vi "standard frame scan geometry_grMD.vi"() -> (3 "frame scan geometry out":waveform(dbl)[](array[waveform]))   [LabVIEW 2017]
doc: "SciScan 1.2 160622"
uses:
  <vilib>/Analysis/coordinate.llb/2D Cartesian Coordinate Rotation (Array).vi
  GFG/GFGnumericGet.vi
  GFG/GFGbooleanGet.vi
  GFG/GFG library.lvlib
  <vilib>/Analysis/NI_AALPro.lvlib
panel:
  out "x waveform":waveform(dbl)
  out "y waveform":waveform(dbl)
  out "Waveform Graph 2":waveform(dbl)(graph)
  out "Waveform Graph":waveform(dbl)(graph)
  out "y waveform (two frames)":dbl[](array[numeric])
  out "x waveform (two frames)":dbl[](array[numeric])
  out "XY Graph":cluster{"Y":dbl[], "Y":dbl[]}[](graph)
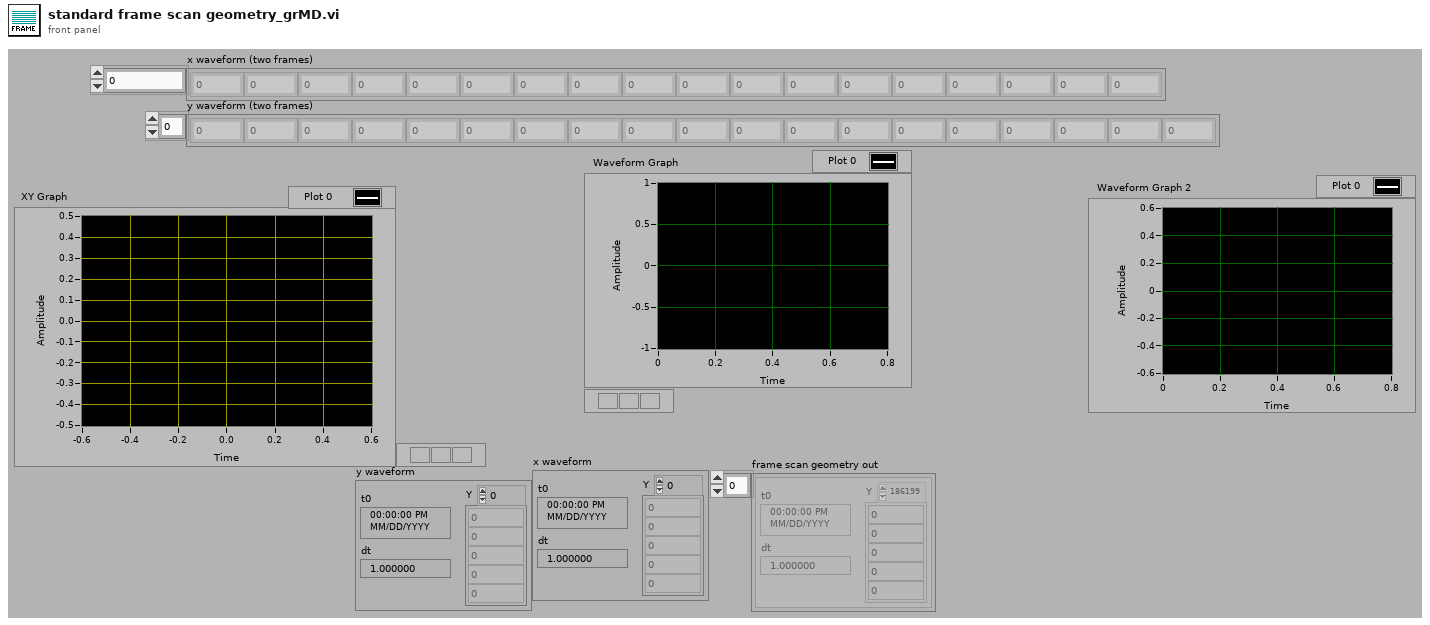
[diagram p1: front panel]
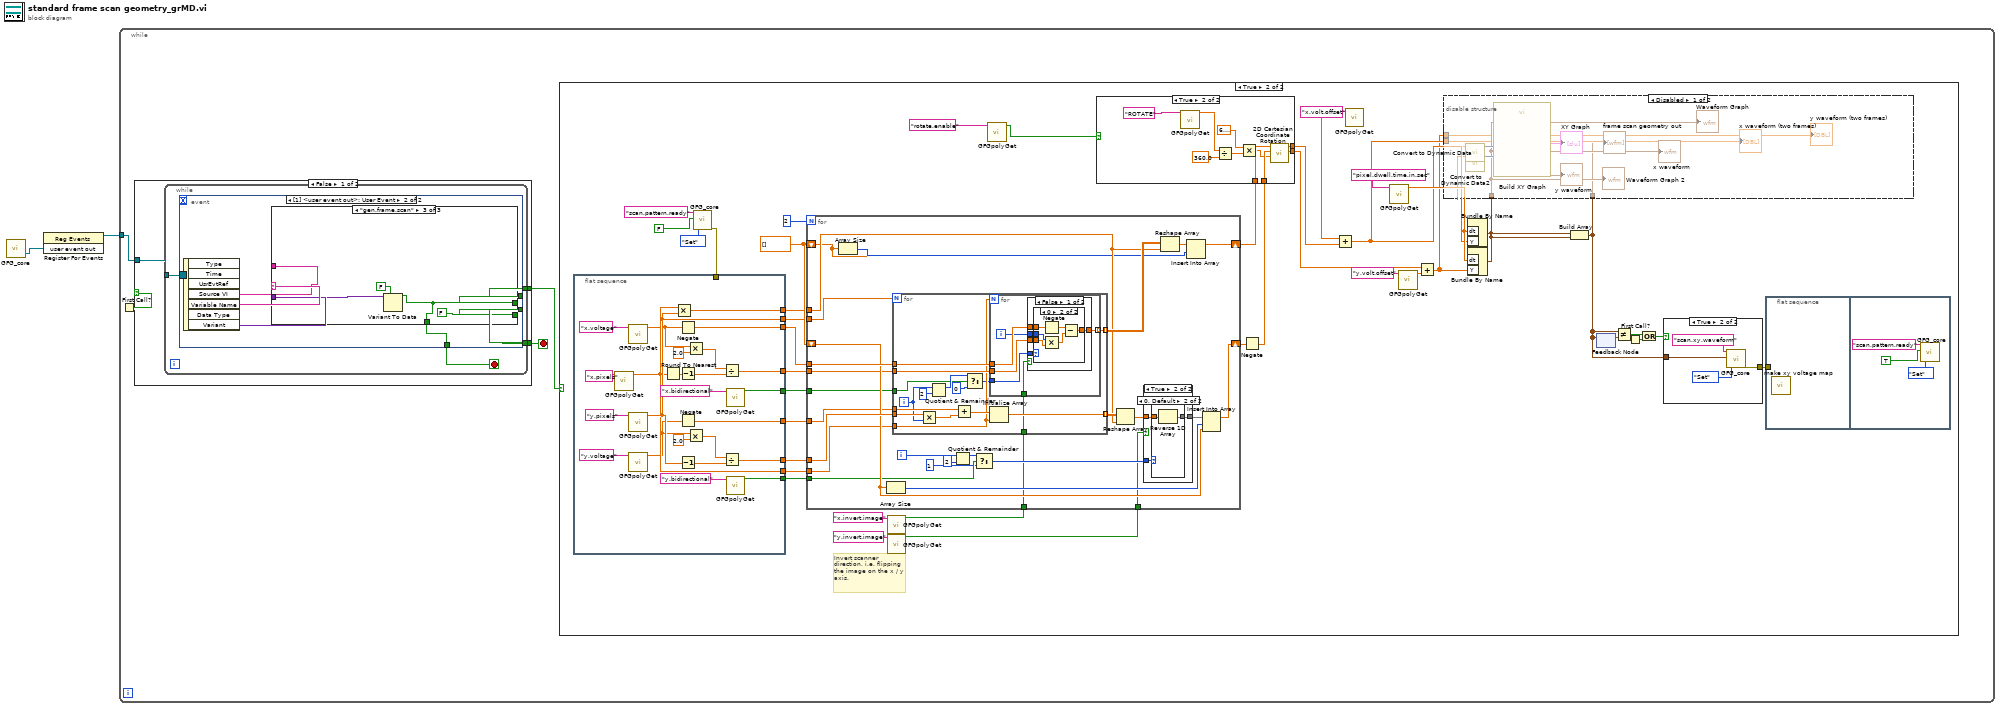
[diagram p0: block diagram]
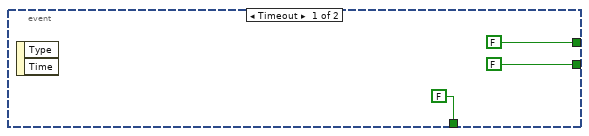
[diagram p2: hidden frame]
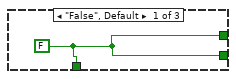
[diagram p3: hidden frame]
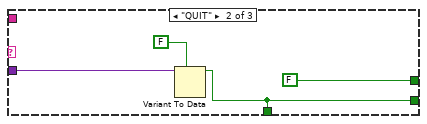
[diagram p4: hidden frame]
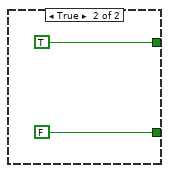
[diagram p5: hidden frame]
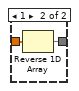
[diagram p11: hidden frame]
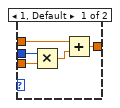
[diagram p13: hidden frame]
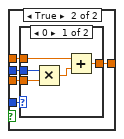
[diagram p14: hidden frame]
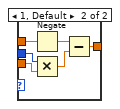
[diagram p15: hidden frame]
diagram:
  n1 = call "GFG_core.vi"() -> ("user event out"=w2:refnum<user-event>)  [unwired: 13 in, 6 out]
  n2 = register-events(w2) -> (reference out=w1:refnum<event-registration>)  [unwired: 2 in, 1 out]
  n3 = while {
    tunnel: w1 -> [w6]
    stop <- w5 stop-if-true
    n4 = First Call?() -> (First Call?: T/F=w3:bool)
    n5 = case shown="False" w3 {
      tunnel: w6 -> [w9 _]
      tunnel: [w8 FALSE ("NewVal")] -> w5
      tunnel: [w7 TRUE ("NewVal")] -> w4
      frame False {
        n6 = while {
          tunnel: w9 -> [w13]
          tunnel: [w11] -> w8
          tunnel: [w12] -> w7
          stop <- w10 stop-if-true
          n7 = event shown="[1] <user event out>: User Event" {
            selector: w13 -> [_ _]
            dyn-events: _ -> [_ _]
            timeout: _ -> [_ _]
            tunnel: [FALSE ("NewVal") w21] -> w12
            tunnel: [FALSE ("NewVal") w20] -> w11
            tunnel: [FALSE w18] -> w10
            event Timeout {
              n8 = event-data() -> ()  [unwired: 1 in, 2 out]
            }
            event User Event {
              n9 = event-data() -> ("Source VI"=w17:string, "Variable Name"=w22:string, "Variant"=w19:variant)  [unwired: 1 in, 4 out]
              n10 = case shown="\"gen.frame.scan\"" w22 {
                tunnel: [w23 FALSE ("NewVal") w28] -> w21
                tunnel: [w23 w24 FALSE] -> w20
                tunnel: w19 -> [_ w27 w29]
                tunnel: [w23 w24 w28] -> w18
                tunnel: w17 -> [_ _ _]
                frame "False", Default {
                  w23 = FALSE ("NewVal")
                }
                frame "QUIT" {
                  n11 = Variant To Data(type=FALSE ("NewVal"), Variant=w27) -> (data=w24:bool)  [unwired: 1 in, 1 out]
                }
                frame "gen.frame.scan" {
                  n12 = Variant To Data(type=FALSE ("NewVal"), Variant=w29) -> (data=w28:bool)  [unwired: 1 in, 1 out]
                }
              }
            }
          }
        }
      }
      frame True {
      }
    }
    n13 = case shown="True" w4 {
      frame False {
      }
      frame True {
        w72 = dbl[] []
        # "Invert scanner direction, i.e. flipping the image on the x / y axis."
        n14 = flat-sequence {
          tunnel: [w109] -> w75
          tunnel: [w108] -> w74
          tunnel: [w106] -> w71
          tunnel: [w102] -> w70
          tunnel: [w101] -> w69
          tunnel: [w100] -> w68
          tunnel: [w98] -> w67
          tunnel: [w92] -> w66
          tunnel: [w90] -> w65
          tunnel: w46 -> [_]
          frame #0 {
            n15 = call-poly "GFGpolyGet.vi"("Variable Name in"="x.pixels" ("Tag in")) -> ("Numeric"=w98:dbl)  [unwired: 8 in, 2 out]
            n16 = call-poly "GFGpolyGet.vi"("Variable Name in"="x.voltage" ("Tag in")) -> ("Numeric"=w96:dbl)  [unwired: 8 in, 2 out]
            n17 = call-poly "GFGpolyGet.vi"("Variable Name in"="y.pixels" ("Tag in")) -> ("Numeric"=w100:dbl)  [unwired: 8 in, 2 out]
            n18 = call-poly "GFGpolyGet.vi"("Variable Name in"="y.voltage" ("Tag in")) -> ("Numeric"=w94:dbl)  [unwired: 8 in, 2 out]
            n19 = Round To Nearest(number=w98) -> (nearest integer value=w88:dbl)
            n20 = Multiply(x=w98, y=w100) -> (x*y=w101:dbl)
            n21 = Negate(x=w96) -> (-x=w109:dbl)
            n22 = Decrement(x=w88) -> (x-1=w105:dbl)
            n23 = Negate(x=w94) -> (-x=w106:dbl)
            n24 = Decrement(x=w100) -> (x-1=w107:dbl)
            n25 = Multiply(x=w96, y=2.0) -> (x*y=w104:dbl)
            n26 = Multiply(x=w94, y=2.0) -> (x*y=w110:dbl)
            n27 = Divide(x=w104, y=w105) -> (x/y=w102:dbl)
            n28 = Divide(x=w110, y=w107) -> (x/y=w108:dbl)
            n29 = call-poly "GFGpolyGet.vi"("Variable Name in"="x.bidirectional" ("Tag in")) -> ("Boolean Value OUT"=w90:bool)  [unwired: 9 in, 1 out]
            n30 = call-poly "GFGpolyGet.vi"("Variable Name in"="y.bidirectional" ("Tag in")) -> ("Boolean Value OUT"=w92:bool)  [unwired: 9 in, 1 out]
          }
        }
        n31 = call "GFG_core.vi"("Variable Name in"="scan.pattern.ready", "Variant in"=FALSE, "Action"=enum16{"Init", "Set", "Get"}."Set") -> ("error out"=w46:errorcluster)  [unwired: 10 in, 6 out]
        n32 = call-poly "GFGpolyGet.vi"("Variable Name in"="x.invert.image" ("Tag in")) -> ("Boolean Value OUT"=w34:bool)  [unwired: 9 in, 1 out]
        n33 = call-poly "GFGpolyGet.vi"("Variable Name in"="y.invert.image" ("Tag in")) -> ("Boolean Value OUT"=w35:bool)  [unwired: 9 in, 1 out]
        n34 = for {
          N: 2 -> [_]
          tunnel: w75 -> [w153]
          tunnel: w74 -> [w152]
          tunnel: w68 -> [w136]
          tunnel: w69 -> [w149]
          shift-right: [w144] -> w38
          shift-left: w72 -> [w146]
          shift-right: [w140] -> w37
          shift-left: w72 -> [w142]
          tunnel: w67 -> [w139]
          tunnel: w71 -> [w138]
          tunnel: w70 -> [w137]
          tunnel: w66 -> [w132]
          tunnel: w65 -> [w131]
          tunnel: w35 -> [w127]
          tunnel: w34 -> [w128]
          i -> [w130]
          n35 = Array Size(array=w146) -> (size(s)=w147:i32)
          n36 = Array Size(array=w142) -> (size(s)=w141:i32)
          n37 = for {
            N: w136 -> [_]
            tunnel: w139 -> [w173]
            tunnel: w153 -> [w175]
            tunnel: w152 -> [w181]
            tunnel: [w178] -> w151 mode=indexing
            tunnel: [w177] -> w150 mode=indexing
            tunnel: w138 -> [w176]
            tunnel: w137 -> [w174]
            tunnel: w131 -> [w167]
            tunnel: w128 -> [w166]
            i -> [w169]
            n38 = Multiply(x=w181, y=w169) -> (x*y=w180:dbl)
            n39 = Quotient & Remainder(x=w169, y=2) -> (x-y*floor(x/y)=w172:i32)  [unwired: 1 out]
            n40 = Add(x=w176, y=w180) -> (x+y=w179:dbl)
            n41 = Select(t=w172, s=w167, f=0) -> (s? t:f=w168:i32)
            n42 = for {
              N: w173 -> [_]
              tunnel: w174 -> [w187]
              tunnel: [w186] -> w178 mode=indexing
              tunnel: w175 -> [w185]
              tunnel: w168 -> [w183]
              tunnel: w166 -> [w182]
              i -> [w184]
              n43 = case shown="False" w182 {
                tunnel: w187 -> [w192 w206]
                tunnel: [w191 w205] -> w186
                tunnel: w185 -> [w190 w208]
                tunnel: w184 -> [w189 w207]
                tunnel: w183 -> [w188 w204]
                frame False {
                  n44 = case shown="0" w188 {
                    tunnel: w192 -> [w197 w203]
                    tunnel: [w196 w202] -> w191
                    tunnel: w190 -> [w195 w201]
                    tunnel: w189 -> [w193 w199]
                    frame 1, Default {
                      n45 = Multiply(x=w193, y=w197) -> (x*y=w194:dbl)
                      n46 = Add(x=w195, y=w194) -> (x+y=w196:dbl)
                    }
                    frame 0 {
                      n47 = Negate(x=w201) -> (-x=w198:dbl)
                      n48 = Multiply(x=w199, y=w203) -> (x*y=w200:dbl)
                      n49 = Subtract(x=w198, y=w200) -> (x-y=w202:dbl)
                    }
                  }
                }
                frame True {
                  n50 = case shown="0" w204 {
                    tunnel: w206 -> [w213 w219]
                    tunnel: [w212 w218] -> w205
                    tunnel: w208 -> [w211 w217]
                    tunnel: w207 -> [w209 w215]
                    frame 0 {
                      n51 = Multiply(x=w209, y=w213) -> (x*y=w210:dbl)
                      n52 = Add(x=w211, y=w210) -> (x+y=w212:dbl)
                    }
                    frame 1, Default {
                      n53 = Negate(x=w217) -> (-x=w214:dbl)
                      n54 = Multiply(x=w215, y=w219) -> (x*y=w216:dbl)
                      n55 = Subtract(x=w214, y=w216) -> (x-y=w218:dbl)
                    }
                  }
                }
              }
            }
            n56 = Initialize Array(w179, w173) -> (w177:dbl[])
          }
          n57 = Quotient & Remainder(x=w130, y=2) -> (x-y*floor(x/y)=w134:i32)  [unwired: 1 out]
          n58 = Select(t=w134, s=w132, f=1) -> (s? t:f=w133:i32)
          n59 = Reshape Array(w150, w149) -> (w148:dbl[])
          n60 = case shown="True" w127 {
            tunnel: w148 -> [w156 w162]
            tunnel: [w155 w161] -> w143
            tunnel: w133 -> [w154 w160]
            frame False {
              n61 = case shown="0, Default" w154 {
                tunnel: [w157 w158] -> w155
                tunnel: w156 -> [w157 w159]
                frame 0, Default {
                }
                frame 1 {
                  n62 = Reverse 1D Array(array=w159) -> (reversed array=w158:dbl[])
                }
              }
            }
            frame True {
              n63 = case shown="0, Default" w160 {
                tunnel: [w163 w164] -> w161
                tunnel: w162 -> [w163 w165]
                frame 1 {
                }
                frame 0, Default {
                  n64 = Reverse 1D Array(array=w165) -> (reversed array=w164:dbl[])
                }
              }
            }
          }
          n65 = Reshape Array(w151, w149) -> (w145:dbl[])
          n66 = Insert Into Array(array=w145, index=w147, new element=w146) -> (w144:dbl[])
          n67 = Insert Into Array(array=w143, index=w141, new element=w142) -> (w140:dbl[])
        }
        n68 = call-poly "GFGpolyGet.vi"("Variable Name in"="rotate.enable" ("Tag in")) -> ("Boolean Value OUT"=w55:bool)  [unwired: 9 in, 1 out]
        n69 = Negate(x=w37) -> (-x=w36:dbl[])
        n70 = case shown="True" w55 {
          tunnel: w38 -> [w115 w126]
          tunnel: w36 -> [w116 w125]
          tunnel: [w115 w118] -> w53
          tunnel: [w116 w117] -> w52
          frame False {
          }
          frame True {
            n71 = call-poly "GFGpolyGet.vi"("Variable Name in"="ROTATE" ("Tag in")) -> ("Numeric"=w120:dbl)  [unwired: 8 in, 2 out]
            n72 = Divide(x=w120, y=360.0) -> (x/y=w121:dbl)
            n73 = Multiply(x=6.283185307179586, y=w121) -> (x*y=w119:dbl)
            n74 = call-poly <vilib>:"2D Cartesian Coordinate Rotation.vi"("theta"=w119, "Y"=w125, "X"=w126) -> ("Y Out"=w117:dbl[], "X Out"=w118:dbl[])  [unwired: 6 in, 1 out]
          }
        }
        n75 = call-poly "GFGpolyGet.vi"("Variable Name in"="x.volt.offset" ("Tag in")) -> ("Numeric"=w62:dbl)  [unwired: 8 in, 2 out]
        n76 = Add(x=w62, y=w53) -> (x+y=w51:dbl[])
        n77 = call-poly "GFGpolyGet.vi"("Variable Name in"="pixel.dwell.time.in.sec" ("Tag in")) -> ("Numeric"=w57:dbl)  [unwired: 8 in, 2 out]
        n78 = call-poly "GFGpolyGet.vi"("Variable Name in"="y.volt.offset" ("Tag in")) -> ("Numeric"=w60:dbl)  [unwired: 8 in, 2 out]
        n79 = Add(x=w52, y=w60) -> (x+y=w50:dbl[])
        n80 = Bundle By Name("dt"=w57, "Y"=w51) -> (w59:waveform(dbl))  [unwired: 1 in]
        n81 = Bundle By Name("dt"=w57, "Y"=w50) -> (w58:waveform(dbl))  [unwired: 1 in]
        n82 = Build Array(w59, w58) -> (w45:waveform(dbl)[])
        n83 = disable-structure shown="Disabled" {
          disable-tunnel: w59 -> [w80 _]
          disable-tunnel: w58 -> [w79 _]
          disable-tunnel: w51 -> [w78 _]
          disable-tunnel: w50 -> [w77 _]
          disable-tunnel: w45 -> [w76 _]
          frame Disabled {
            n84 = call "Convert to Dynamic Data"("Array"=w78) -> ("Dynamic Data Type"=w82:dynamicdata)  [unwired: 3 in]
            n85 = call "Convert to Dynamic Data2"("Array"=w77) -> ("Dynamic Data Type"=w81:dynamicdata)  [unwired: 3 in]
            n86 = call "Build XY Graph"("Y Input"=w81, "X Input"=w82) -> ("XY Graph"=→"XY Graph":cluster{"Y":dbl[], "Y":dbl[]}[])  [unwired: 8 in, 1 out]
            "x waveform (two frames)" <- w78
            "y waveform (two frames)" <- w77
            "Waveform Graph" <- w80
            "Waveform Graph 2" <- w79
            "y waveform" <- w79
            "x waveform" <- w80
            "frame scan geometry out" <- w76
          }
          frame Enabled {
          }
        }
        n87 = feedback-in #1(w45) -> ()
        n88 = feedback #1() -> (w44:waveform(dbl)[])  [unwired: 1 in]
        n89 = Not Equal?(x=w45, y=w44) -> (x != y?=w43:bool)
        n90 = First Call?() -> (First Call?: T/F=w41:bool)
        n91 = Or(x=w43, y=w41) -> (x .or. y?=w42:bool)
        n92 = case shown="True" w42 {
          tunnel: w45 -> [_ w86]
          tunnel: [_ w84] -> w54
          frame False {
          }
          frame True {
            n93 = call "GFG_core.vi"("Variable Name in"="scan.xy.waveform", "Variant in"=w86, "Action"=enum16{"Init", "Set", "Get"}."Set") -> ("error out"=w84:errorcluster)  [unwired: 10 in, 6 out]
          }
        }
        n94 = flat-sequence {
          tunnel: w54 -> [_]
          frame #0 {
            n95 = call "make xy voltage map.vi"() -> ()  [unwired: 12 in]
          }
          frame #1 {
            n96 = call "GFG_core.vi"("Variable Name in"="scan.pattern.ready", "Variant in"=TRUE, "Action"=enum16{"Init", "Set", "Get"}."Set") -> ()  [unwired: 10 in, 7 out]
          }
        }
      }
    }
  }
